vi "ChangeColor.vi"() -> ()   [LabVIEW 2013]
doc: "This VI show how to change backgound color of multilist box control active cell ."
uses:
  <vilib>/Utility/miscctls.llb/LVRowAndColumnTypeDef.ctl
  <vilib>/Utility/miscctls.llb/LVBoundsTypeDef.ctl
panel:
  in  "Multicolumn Listbox":i32(listbox)
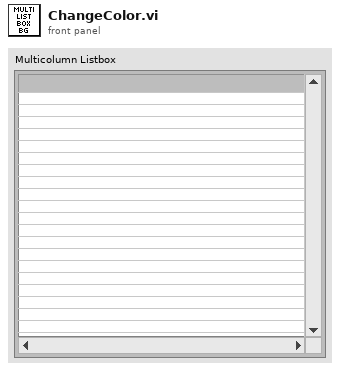
[diagram p1: front panel]
types:
  T1 = typedef "LVBoundsTypeDef.ctl" = cluster{"Width":u32, "Height":u32}
  T2 = typedef "LVRowAndColumnTypeDef.ctl" = cluster{"Row":i32, "Column":i32}
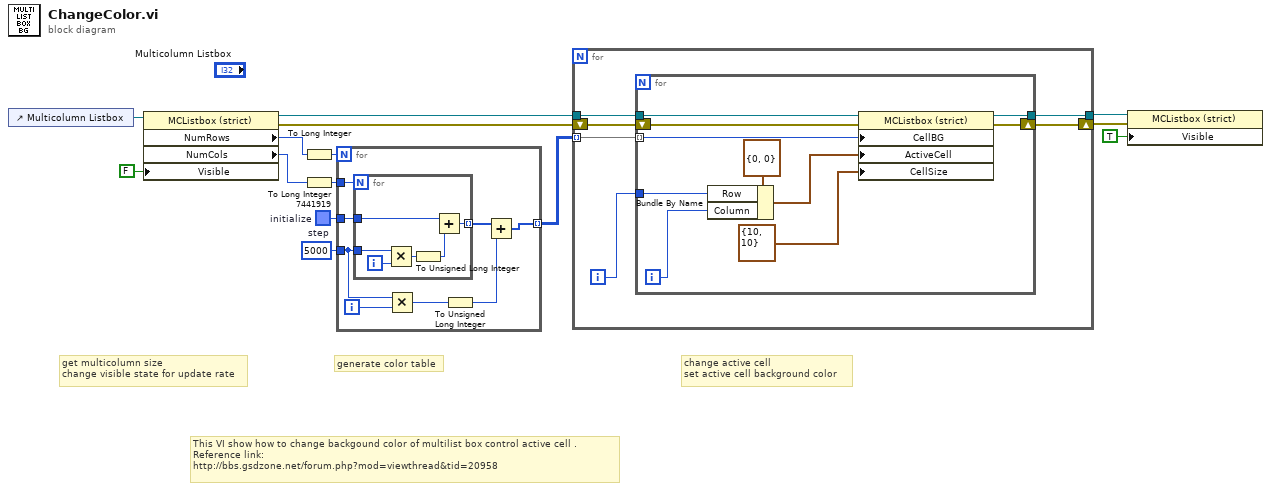
[diagram p0: block diagram]
diagram:
  w7 = 5000  # step
  w10 = u32 7441919  # initialize
  # "This VI show how to change backgound color of multilist box control active cell .\nReference link: \nhttp://bbs.gsdzone.net/forum.php?mod=viewthread&tid=20958"
  # "get multicolumn size\nchange visible state for update rate"
  # "change active cell\nset active cell background color"
  # "generate color table"
  n1 = control-ref of="Multicolumn Listbox"() -> (w14:refnum<vi>)
  n2 = property class="MCListbox (strict)"(reference=w14, "Visible"=FALSE) -> (reference out=w13:refnum<vi>, error out=w12:errorcluster, "NumRows"=w9:u32, "NumCols"=w8:u32)  [unwired: 1 in]
  n3 = To Long Integer(number=w9) -> (32bit integer=w2:i32)
  n4 = To Long Integer(number=w8) -> (32bit integer=w1:i32)
  n5 = for {
    N: w2 -> [_]
    tunnel: w1 -> [w22]
    tunnel: [w17] -> w11 mode=indexing
    tunnel: w10 -> [w21]
    tunnel: w7 -> [w16]
    i -> [w20]
    n6 = for {
      N: w22 -> [_]
      tunnel: w21 -> [w26]
      tunnel: [w25] -> w18 mode=indexing
      tunnel: w16 -> [w24]
      i -> [w28]
      n7 = Multiply(x=w24, y=w28) -> (x*y=w27:i32)
      n8 = To Unsigned Long Integer(number=w27) -> (unsigned 32bit integer=w23:u32)
      n9 = Add(x=w26, y=w23) -> (x+y=w25:u32)
    }
    n10 = Multiply(x=w16, y=w20) -> (x*y=w19:i32)
    n11 = To Unsigned Long Integer(number=w19) -> (unsigned 32bit integer=w15:u32)
    n12 = Add(x=w18, y=w15) -> (x+y=w17:u32[])
  }
  n13 = for {
    tunnel: w13 -> [w34]
    tunnel: w11 -> [w32] mode=indexing
    shift-right: [w30] -> w4
    shift-left: w12 -> [w33]
    tunnel: [w29] -> w5
    i -> [w31]
    n14 = for {
      tunnel: w34 -> [w44]
      tunnel: w32 -> [w42] mode=indexing
      tunnel: w31 -> [w38]
      shift-right: [w36] -> w30
      shift-left: w33 -> [w43]
      tunnel: [w35] -> w29
      i -> [w39]
      n15 = Bundle By Name(cluster=T2 {"Row"=0, "Column"=0} ("Active Cell:Active Cell"), "Row"=w38, "Column"=w39) -> (w40:T2)
      n16 = property class="MCListbox (strict)"(reference=w44, error in=w43, "CellBG"=w42, "ActiveCell"=w40, "CellSize"=T1 {"Width"=10, "Height"=10} ("Active Cell:Cell Size")) -> (reference out=w35:refnum<vi>, error out=w36:errorcluster)
    }
  }
  n17 = property class="MCListbox (strict)"(reference=w5, error in=w4, "Visible"=TRUE) -> ()  [unwired: 2 out]
